vi "Lab Panel V5.31.vi"() -> ()   [LabVIEW 2017] (continued)
                            n1476 = local write "RESULT LAB04-1"(TRUE) -> ()
                            n1477 = local write "DISP LAB04-1"(w2766) -> ()
                          }
                        }
                      }
                      frame False {
                      }
                    }
                  }
                }
              }
              frame #7 {
                # "LAB04-2"
                n1478 = Equal?(x=w2769, y=2) -> (x = y?=w2772:bool)
                n1479 = local read "DISP LAB04-2"() -> (w2774:T4)
                n1480 = Unbundle(w2774) -> ("STATUS"=w2775:string)  [unwired: 2 out]
                n1481 = Equal?(x=w2775, y="RUN") -> (x = y?=w2771:bool)
                n1482 = And(x=w2771, y=w2772) -> (x .and. y?=w2770:bool)
                n1483 = case shown="True" w2770 {
                  tunnel: w2774 -> [_ w2778]
                  tunnel: w2768 -> [_ w2781]
                  frame False {
                  }
                  frame True {
                    n1484 = local read "SET LAB04-2"() -> (w2780:T5)
                    n1485 = local read "TDMS LAB04-2"() -> (w2777:refnum<k34>)
                    n1486 = Unbundle(w2778) -> ("CYCLE"=w2782:dbl)  [unwired: 2 out]
                    n1487 = Unbundle(w2780) -> ("T-RISE mins"=w2779:dbl)  [unwired: 4 out]
                    n1488 = Greater Or Equal?(x=w2782, y=w2781) -> (x >= y?=w2783:bool)
                    n1489 = case shown="True" w2783 {
                      tunnel: w2779 -> [w2786 _]
                      tunnel: w2778 -> [w2785 _]
                      tunnel: w2777 -> [w2784 _]
                      frame True {
                        n1490 = stacked-sequence {
                          tunnel: w2786 -> [w2789 _]
                          tunnel: w2785 -> [_ w2794]
                          tunnel: w2784 -> [w2787 _]
                          frame #0 {
                            n1491 = Build Array("T-RISE") -> (w2791:string[])
                            n1492 = Build Array(w2789) -> (w2790:dbl[])
                            n1493 = TDMS Write(0:w2787, 5:"TEST PASS", 7:w2791, 9:w2790) -> (15:w2793:errorcluster)  [unwired: 2 in, 3 out]
                            n1494 = local write "data file error"(w2793) -> ()
                          }
                          frame #1 {
                            n1495 = Bundle(cluster=w2794, "STATUS"="T-RISE PASS") -> (w2796:T4)  [unwired: 2 in]
                            n1496 = local write "RESULT LAB04-2"(TRUE) -> ()
                            n1497 = local write "DISP LAB04-2"(w2796) -> ()
                          }
                        }
                      }
                      frame False {
                      }
                    }
                  }
                }
              }
              frame #8 {
                # "LAB05-1"
                n1498 = Equal?(x=w2799, y=2) -> (x = y?=w2802:bool)
                n1499 = local read "DISP LAB05-1"() -> (w2804:T4)
                n1500 = Unbundle(w2804) -> ("STATUS"=w2805:string)  [unwired: 2 out]
                n1501 = Equal?(x=w2805, y="RUN") -> (x = y?=w2801:bool)
                n1502 = And(x=w2801, y=w2802) -> (x .and. y?=w2800:bool)
                n1503 = case shown="True" w2800 {
                  tunnel: w2804 -> [_ w2808]
                  tunnel: w2798 -> [_ w2811]
                  frame False {
                  }
                  frame True {
                    n1504 = local read "SET LAB05-1"() -> (w2810:T5)
                    n1505 = local read "TDMS LAB05-1"() -> (w2807:refnum<k34>)
                    n1506 = Unbundle(w2808) -> ("CYCLE"=w2812:dbl)  [unwired: 2 out]
                    n1507 = Unbundle(w2810) -> ("T-RISE mins"=w2809:dbl)  [unwired: 4 out]
                    n1508 = Greater Or Equal?(x=w2812, y=w2811) -> (x >= y?=w2813:bool)
                    n1509 = case shown="True" w2813 {
                      tunnel: w2809 -> [w2816 _]
                      tunnel: w2808 -> [w2815 _]
                      tunnel: w2807 -> [w2814 _]
                      frame True {
                        n1510 = stacked-sequence {
                          tunnel: w2816 -> [w2819 _]
                          tunnel: w2815 -> [_ w2824]
                          tunnel: w2814 -> [w2817 _]
                          frame #0 {
                            n1511 = Build Array("T-RISE") -> (w2821:string[])
                            n1512 = Build Array(w2819) -> (w2820:dbl[])
                            n1513 = TDMS Write(0:w2817, 5:"TEST PASS", 7:w2821, 9:w2820) -> (15:w2823:errorcluster)  [unwired: 2 in, 3 out]
                            n1514 = local write "data file error"(w2823) -> ()
                          }
                          frame #1 {
                            n1515 = Bundle(cluster=w2824, "STATUS"="T-RISE PASS") -> (w2826:T4)  [unwired: 2 in]
                            n1516 = local write "RESULT LAB05-1"(TRUE) -> ()
                            n1517 = local write "DISP LAB05-1"(w2826) -> ()
                          }
                        }
                      }
                      frame False {
                      }
                    }
                  }
                }
              }
              frame #9 {
                # "LAB05-2"
                n1518 = Equal?(x=w2829, y=2) -> (x = y?=w2832:bool)
                n1519 = local read "DISP LAB05-2"() -> (w2834:T4)
                n1520 = Unbundle(w2834) -> ("STATUS"=w2835:string)  [unwired: 2 out]
                n1521 = Equal?(x=w2835, y="RUN") -> (x = y?=w2831:bool)
                n1522 = And(x=w2831, y=w2832) -> (x .and. y?=w2830:bool)
                n1523 = case shown="True" w2830 {
                  tunnel: w2834 -> [_ w2838]
                  tunnel: w2828 -> [_ w2841]
                  frame False {
                  }
                  frame True {
                    n1524 = local read "SET LAB05-2"() -> (w2840:T5)
                    n1525 = local read "TDMS LAB05-2"() -> (w2837:refnum<k34>)
                    n1526 = Unbundle(w2838) -> ("CYCLE"=w2842:dbl)  [unwired: 2 out]
                    n1527 = Unbundle(w2840) -> ("T-RISE mins"=w2839:dbl)  [unwired: 4 out]
                    n1528 = Greater Or Equal?(x=w2842, y=w2841) -> (x >= y?=w2843:bool)
                    n1529 = case shown="True" w2843 {
                      tunnel: w2839 -> [w2846 _]
                      tunnel: w2838 -> [w2845 _]
                      tunnel: w2837 -> [w2844 _]
                      frame True {
                        n1530 = stacked-sequence {
                          tunnel: w2846 -> [w2849 _]
                          tunnel: w2845 -> [_ w2854]
                          tunnel: w2844 -> [w2847 _]
                          frame #0 {
                            n1531 = Build Array("T-RISE") -> (w2851:string[])
                            n1532 = Build Array(w2849) -> (w2850:dbl[])
                            n1533 = TDMS Write(0:w2847, 5:"TEST PASS", 7:w2851, 9:w2850) -> (15:w2853:errorcluster)  [unwired: 2 in, 3 out]
                            n1534 = local write "data file error"(w2853) -> ()
                          }
                          frame #1 {
                            n1535 = Bundle(cluster=w2854, "STATUS"="T-RISE PASS") -> (w2856:T4)  [unwired: 2 in]
                            n1536 = local write "RESULT LAB05-2"(TRUE) -> ()
                            n1537 = local write "DISP LAB05-2"(w2856) -> ()
                          }
                        }
                      }
                      frame False {
                      }
                    }
                  }
                }
              }
            }
          }
          frame #7 {
            # "Note : run lab0X-N. RUN LAB0X-N and O/I LAB0X-N   are written to digital I/O in frame 11"
            # "End test & close test files"
            n1538 = local read "MAIL SETTINGS"() -> (w2863:T8)
            n1539 = local read "TO (string):"() -> (w2858:string)
            n1540 = Unbundle(w2863) -> ("OUT SERVER ADDRESS"=w2862:string, "FROM ACCOUNT"=w2861:string)  [unwired: 5 out]
            n1541 = stacked-sequence {
              tunnel: w2873 -> [_ _ _ _ _ _ _ _ _ _]
              tunnel: w2874 -> [_ _ _ _ _ _ _ _ _ _]
              tunnel: w2872 -> [_ _ _ _ _ _ _ _ _ _]
              tunnel: w2871 -> [_ _ _ _ _ _ _ _ _ _]
              tunnel: w2870 -> [_ _ _ _ _ _ _ _ _ _]
              tunnel: w2869 -> [_ _ _ _ _ _ _ _ _ _]
              tunnel: w2868 -> [_ _ _ _ _ _ _ _ _ _]
              tunnel: w2867 -> [_ _ _ _ _ _ _ _ _ _]
              tunnel: w2866 -> [_ _ _ _ _ _ _ _ _ _]
              tunnel: w2865 -> [_ _ _ _ _ _ _ _ _ _]
              tunnel: w2862 -> [w2879 w2931 w2979 w3026 w3073 w3120 w3167 w3214 w3261 w3308]
              tunnel: w2861 -> [w2878 w2930 w2978 w3025 w3072 w3119 w3166 w3213 w3260 w3307]
              tunnel: "Mail Test File To:" -> [w2877 w2929 w2977 w3024 w3071 w3118 w3165 w3212 w3259 w3306]
              tunnel: "Mail Test Fail" -> [w2876 w2928 w2976 w3023 w3070 w3117 w3164 w3211 w3258 w3305]
              frame #0 {
                # "LAB01-1"
                n1542 = local read "DISP LAB01-1"() -> (w2875:T4)
                n1543 = global write "Global display 2.vi" "DISP LAB01-1"(w2875) -> ()
                n1544 = local read "run lab01-1"() -> (w2880:bool)
                n1545 = local read "TDMS LAB01-1"() -> (w2881:refnum<k34>)
                n1546 = Unbundle(w2875) -> ("CYCLE"=w2883:dbl, "STATUS"=w2882:string)  [unwired: 1 out]
                n1547 = case shown="True" w2880 {
                  tunnel: w2883 -> [_ w2889]
                  tunnel: w2875 -> [_ w2891]
                  tunnel: w2882 -> [_ w2888]
                  tunnel: w2881 -> [_ w2890]
                  tunnel: w2879 -> [_ w2887]
                  tunnel: w2878 -> [_ w2886]
                  tunnel: w2877 -> [_ w2885]
                  tunnel: w2876 -> [_ w2884]
                  frame False {
                  }
                  frame True {
                    n1548 = Not Equal?(x=w2888, y="RUN") -> (x != y?=w2892:bool)
                    n1549 = Greater?(x=w2889, y=2.0) -> (0:w2894:bool)
                    n1550 = And(x=w2894, y=w2892) -> (x .and. y?=w2893:bool)
                    n1551 = case shown="True" w2893 {
                      tunnel: w2891 -> [_ w2904]
                      tunnel: w2890 -> [_ w2903]
                      tunnel: w2889 -> [_ w2902]
                      tunnel: w2888 -> [_ w2901]
                      tunnel: w2887 -> [_ w2900]
                      tunnel: w2886 -> [_ w2899]
                      tunnel: w2885 -> [_ w2898]
                      tunnel: w2884 -> [_ w2897]
                      frame False {
                      }
                      frame True {
                        n1552 = stacked-sequence {
                          tunnel: w2904 -> [w2908 _ _]
                          tunnel: w2903 -> [_ w2910 _]
                          tunnel: w2902 -> [_ _ _]
                          tunnel: w2901 -> [_ _ w2916]
                          tunnel: w2900 -> [_ _ w2915]
                          tunnel: w2899 -> [_ _ w2914]
                          tunnel: w2898 -> [_ _ w2913]
                          tunnel: w2897 -> [_ _ w2912]
                          frame #0 {
                            w2905 = FALSE
                            n1553 = local write "mail control"("END") -> ()
                            n1554 = Bundle(cluster=w2908) -> (w2907:T4)  [unwired: 3 in]
                            n1555 = local write "DISP LAB01-1"(w2907) -> ()
                            n1556 = local write "O/I  LAB01-1"(w2905) -> ()
                            n1557 = local write "run lab01-1"(w2905) -> ()
                            n1558 = local write "RUN LAB01-1"(w2905) -> ()
                          }
                          frame #1 {
                            n1559 = TDMS Close(11:w2910) -> (0:w2909:errorcluster)  [unwired: 1 in, 1 out]
                            n1560 = local write "data file error"(w2909) -> ()
                          }
                          frame #2 {
                            n1561 = stacked-sequence {
                              tunnel: "LAB01-1" -> [w2918 w2921 _]
                              tunnel: w2916 -> [_ w2927 _]
                              tunnel: w2915 -> [_ w2926 _]
                              tunnel: w2914 -> [_ w2925 _]
                              tunnel: w2913 -> [_ w2924 _]
                              tunnel: w2912 -> [_ w2923 _]
                              frame #0 {
                                n1562 = call "sub vi - defrag tdms v1.vi"("panel id"=w2918) -> ("error out"=w2917:errorcluster)  [unwired: 10 in]
                                n1563 = local write "data file error"(w2917) -> ()
                              }
                              frame #1 {
                                n1564 = Bundle By Name(cluster=T23 {"status"="", "mail server"="", "mail from"="", "mail to"="", "mail file"=FALSE} ("Input Cluster"), "status"=w2927, "mail server"=w2926, "mail from"=w2925, "mail to"=w2924, "mail file"=w2923) -> (w2920:T23)
                                n1565 = call "Save data file (pass-fail) v5.vi"("Input Cluster"=w2920, "panel id"=w2921) -> ("network file save error"=w2922:errorcluster)  [unwired: 8 in, 1 out]
                                n1566 = local write "data file error"(w2922) -> ()
                              }
                              frame #2 {
                              }
                            }
                          }
                        }
                      }
                    }
                  }
                }
              }
              frame #1 {
                # "LAB01-2"
                n1567 = local read "run lab01-2"() -> (w2932:bool)
                n1568 = case shown="True" w2932 {
                  tunnel: w2931 -> [_ w2937]
                  tunnel: w2930 -> [_ w2936]
                  tunnel: w2929 -> [_ w2935]
                  tunnel: w2928 -> [_ w2934]
                  frame False {
                  }
                  frame True {
                    n1569 = local read "DISP LAB01-2"() -> (w2933:T4)
                    n1570 = global write "Global display 2.vi" "DISP LAB01-2"(w2933) -> ()
                    n1571 = local read "TDMS LAB01-2"() -> (w2944:refnum<k34>)
                    n1572 = Unbundle(w2933) -> ("CYCLE"=w2939:dbl, "STATUS"=w2938:string)  [unwired: 1 out]
                    n1573 = Not Equal?(x=w2938, y="RUN") -> (x != y?=w2941:bool)
                    n1574 = Greater?(x=w2939, y=2.0) -> (0:w2942:bool)
                    n1575 = And(x=w2942, y=w2941) -> (x .and. y?=w2940:bool)
                    n1576 = case shown="True" w2940 {
                      tunnel: w2933 -> [_ w2953]
                      tunnel: w2944 -> [_ w2952]
                      tunnel: w2939 -> [_ w2951]
                      tunnel: w2938 -> [_ w2950]
                      tunnel: w2937 -> [_ w2949]
                      tunnel: w2936 -> [_ w2948]
                      tunnel: w2935 -> [_ w2947]
                      tunnel: w2934 -> [_ w2946]
                      frame False {
                      }
                      frame True {
                        n1577 = stacked-sequence {
                          tunnel: w2953 -> [w2956 _ _]
                          tunnel: w2952 -> [_ w2958 _]
                          tunnel: w2951 -> [_ _ _]
                          tunnel: w2950 -> [_ _ w2964]
                          tunnel: w2949 -> [_ _ w2963]
                          tunnel: w2948 -> [_ _ w2962]
                          tunnel: w2947 -> [_ _ w2961]
                          tunnel: w2946 -> [_ _ w2960]
                          frame #0 {
                            w2954 = FALSE
                            n1578 = local write "mail control"("END") -> ()
                            n1579 = Bundle(cluster=w2956) -> (w2957:T4)  [unwired: 3 in]
                            n1580 = local write "RUN LAB01-2"(w2954) -> ()
                            n1581 = local write "run lab01-2"(w2954) -> ()
                            n1582 = local write "O/I  LAB01-2"(w2954) -> ()
                            n1583 = local write "DISP LAB01-2"(w2957) -> ()
                          }
                          frame #1 {
                            n1584 = TDMS Close(11:w2958) -> (0:w2959:errorcluster)  [unwired: 1 in, 1 out]
                            n1585 = local write "data file error"(w2959) -> ()
                          }
                          frame #2 {
                            n1586 = stacked-sequence {
                              tunnel: "LAB01-2" -> [w2967 w2968]
                              tunnel: w2964 -> [_ w2973]
                              tunnel: w2963 -> [_ w2972]
                              tunnel: w2962 -> [_ w2971]
                              tunnel: w2961 -> [_ w2970]
                              tunnel: w2960 -> [_ w2969]
                              frame #0 {
                                n1587 = call "sub vi - defrag tdms v1.vi"("panel id"=w2967) -> ("error out"=w2966:errorcluster)  [unwired: 10 in]
                                n1588 = local write "data file error"(w2966) -> ()
                              }
                              frame #1 {
                                n1589 = Bundle("STATUS"=w2973, "OUT SERVER ADDRESS"=w2972, "FROM ACCOUNT"=w2971, "Mail Test File To:"=w2970, "Mail Test Fail"=w2969) -> (w2975:T29)  [unwired: 1 in]
                                n1590 = call "Save data file (pass-fail) v5.vi"("Input Cluster"=w2975, "panel id"=w2968) -> ("network file save error"=w2974:errorcluster)  [unwired: 8 in, 1 out]
                                n1591 = local write "data file error"(w2974) -> ()
                              }
                            }
                          }
                        }
                      }
                    }
                  }
                }
              }
              frame #2 {
                # "LAB02-1"
                n1592 = local read "run lab02-1"() -> (w2980:bool)
                n1593 = case shown="True" w2980 {
                  tunnel: w2979 -> [_ w2985]
                  tunnel: w2978 -> [_ w2984]
                  tunnel: w2977 -> [_ w2983]
                  tunnel: w2976 -> [_ w2982]
                  frame False {
                  }
                  frame True {
                    n1594 = local read "DISP LAB02-1"() -> (w2981:T4)
                    n1595 = global write "Global display 2.vi" "DISP LAB02-1"(w2981) -> ()
                    n1596 = Unbundle(w2981) -> ("CYCLE"=w2989:dbl, "STATUS"=w2986:string)  [unwired: 1 out]
                    n1597 = local read "TDMS LAB02-1"() -> (w2992:refnum<k34>)
                    n1598 = Not Equal?(x=w2986, y="RUN") -> (x != y?=w2988:bool)
                    n1599 = Greater?(x=w2989, y=2.0) -> (0:w2990:bool)
                    n1600 = And(x=w2990, y=w2988) -> (x .and. y?=w2987:bool)
                    n1601 = case shown="True" w2987 {
                      tunnel: w2981 -> [_ w3000]
                      tunnel: w2992 -> [_ w2999]
                      tunnel: w2986 -> [_ w2998]
                      tunnel: w2985 -> [_ w2997]
                      tunnel: w2984 -> [_ w2996]
                      tunnel: w2983 -> [_ w2995]
                      tunnel: w2982 -> [_ w2994]
                      frame False {
                      }
                      frame True {
                        n1602 = stacked-sequence {
                          tunnel: w3000 -> [w3003 _ _]
                          tunnel: w2999 -> [_ w3005 _]
                          tunnel: w2998 -> [_ _ w3011]
                          tunnel: w2997 -> [_ _ w3010]
                          tunnel: w2996 -> [_ _ w3009]
                          tunnel: w2995 -> [_ _ w3008]
                          tunnel: w2994 -> [_ _ w3007]
                          frame #0 {
                            w3001 = FALSE
                            n1603 = local write "mail control"("END") -> ()
                            n1604 = Bundle(cluster=w3003) -> (w3004:T4)  [unwired: 3 in]
                            n1605 = local write "O/I  LAB02-1"(w3001) -> ()
                            n1606 = local write "RUN LAB02-1"(w3001) -> ()
                            n1607 = local write "run lab02-1"(w3001) -> ()
                            n1608 = local write "DISP LAB02-1"(w3004) -> ()
                          }
                          frame #1 {
                            n1609 = TDMS Close(11:w3005) -> (0:w3006:errorcluster)  [unwired: 1 in, 1 out]
                            n1610 = local write "data file error"(w3006) -> ()
                          }
                          frame #2 {
                            n1611 = stacked-sequence {
                              tunnel: "LAB02-1" -> [w3014 w3021]
                              tunnel: w3011 -> [_ w3019]
                              tunnel: w3010 -> [_ w3018]
                              tunnel: w3009 -> [_ w3017]
                              tunnel: w3008 -> [_ w3016]
                              tunnel: w3007 -> [_ w3015]
                              frame #0 {
                                n1612 = call "sub vi - defrag tdms v1.vi"("panel id"=w3014) -> ("error out"=w3013:errorcluster)  [unwired: 10 in]
                                n1613 = local write "data file error"(w3013) -> ()
                              }
                              frame #1 {
                                n1614 = Bundle("STATUS"=w3019, "OUT SERVER ADDRESS"=w3018, "FROM ACCOUNT"=w3017, "Mail Test File To:"=w3016, "Mail Test Fail"=w3015) -> (w3020:T29)  [unwired: 1 in]
                                n1615 = call "Save data file (pass-fail) v5.vi"("Input Cluster"=w3020, "panel id"=w3021) -> ("network file save error"=w3022:errorcluster)  [unwired: 8 in, 1 out]
                                n1616 = local write "data file error"(w3022) -> ()
                              }
                            }
                          }
                        }
                      }
                    }
                  }
                }
              }
              frame #3 {
                # "LAB02-2"
                n1617 = local read "run lab02-2"() -> (w3027:bool)
                n1618 = case shown="True" w3027 {
                  tunnel: w3026 -> [_ w3033]
                  tunnel: w3025 -> [_ w3032]
                  tunnel: w3024 -> [_ w3031]
                  tunnel: w3023 -> [_ w3030]
                  frame False {
                  }
                  frame True {
                    n1619 = local read "DISP LAB02-2"() -> (w3029:T4)
                    n1620 = global write "Global display 2.vi" "DISP LAB02-2"(w3029) -> ()
                    n1621 = local read "TDMS LAB02-2"() -> (w3039:refnum<k34>)
                    n1622 = Unbundle(w3029) -> ("CYCLE"=w3028:dbl, "STATUS"=w3034:string)  [unwired: 1 out]
                    n1623 = Not Equal?(x=w3034, y="RUN") -> (x != y?=w3036:bool)
                    n1624 = Greater?(x=w3028, y=2.0) -> (0:w3037:bool)
                    n1625 = And(x=w3037, y=w3036) -> (x .and. y?=w3035:bool)
                    n1626 = case shown="True" w3035 {
                      tunnel: w3029 -> [_ w3047]
                      tunnel: w3039 -> [_ w3046]
                      tunnel: w3034 -> [_ w3045]
                      tunnel: w3033 -> [_ w3044]
                      tunnel: w3032 -> [_ w3043]
                      tunnel: w3031 -> [_ w3042]
                      tunnel: w3030 -> [_ w3041]
                      frame False {
                      }
                      frame True {
                        n1627 = stacked-sequence {
                          tunnel: w3047 -> [w3050 _ _]
                          tunnel: w3046 -> [_ w3052 _]
                          tunnel: w3045 -> [_ _ w3058]
                          tunnel: w3044 -> [_ _ w3057]
                          tunnel: w3043 -> [_ _ w3056]
                          tunnel: w3042 -> [_ _ w3055]
                          tunnel: w3041 -> [_ _ w3054]
                          frame #0 {
                            w3048 = FALSE
                            n1628 = local write "mail control"("END") -> ()
                            n1629 = Bundle(cluster=w3050) -> (w3051:T4)  [unwired: 3 in]
                            n1630 = local write "O/I  LAB02-2"(w3048) -> ()
                            n1631 = local write "run lab02-2"(w3048) -> ()
                            n1632 = local write "RUN LAB02-2"(w3048) -> ()
                            n1633 = local write "DISP LAB02-2"(w3051) -> ()
                          }
                          frame #1 {
                            n1634 = TDMS Close(11:w3052) -> (0:w3053:errorcluster)  [unwired: 1 in, 1 out]
                            n1635 = local write "data file error"(w3053) -> ()
                          }
                          frame #2 {
                            n1636 = stacked-sequence {
                              tunnel: "LAB02-2" -> [w3061 w3067]
                              tunnel: w3058 -> [_ w3066]
                              tunnel: w3057 -> [_ w3065]
                              tunnel: w3056 -> [_ w3064]
                              tunnel: w3055 -> [_ w3063]
                              tunnel: w3054 -> [_ w3062]
                              frame #0 {
                                n1637 = call "sub vi - defrag tdms v1.vi"("panel id"=w3061) -> ("error out"=w3060:errorcluster)  [unwired: 10 in]
                                n1638 = local write "data file error"(w3060) -> ()
                              }
                              frame #1 {
                                n1639 = Bundle("STATUS"=w3066, "OUT SERVER ADDRESS"=w3065, "FROM ACCOUNT"=w3064, "Mail Test File To:"=w3063, "Mail Test Fail"=w3062) -> (w3069:T29)  [unwired: 1 in]
                                n1640 = call "Save data file (pass-fail) v5.vi"("Input Cluster"=w3069, "panel id"=w3067) -> ("network file save error"=w3068:errorcluster)  [unwired: 8 in, 1 out]
                                n1641 = local write "data file error"(w3068) -> ()
                              }
                            }
                          }
                        }
                      }
                    }
                  }
                }
              }
              frame #4 {
                # "LAB03-1"
                n1642 = local read "run lab03-1"() -> (w3074:bool)
                n1643 = case shown="True" w3074 {
                  tunnel: w3073 -> [_ w3079]
                  tunnel: w3072 -> [_ w3078]
                  tunnel: w3071 -> [_ w3077]
                  tunnel: w3070 -> [_ w3076]
                  frame False {
                  }
                  frame True {
                    n1644 = local read "DISP LAB03-1"() -> (w3075:T4)
                    n1645 = local read "TDMS LAB03-1"() -> (w3086:refnum<k34>)
                    n1646 = global write "Global display 2.vi" "DISP LAB03-1"(w3075) -> ()
                    n1647 = Unbundle(w3075) -> ("CYCLE"=w3083:dbl, "STATUS"=w3080:string)  [unwired: 1 out]
                    n1648 = Not Equal?(x=w3080, y="RUN") -> (x != y?=w3082:bool)
                    n1649 = Greater?(x=w3083, y=2.0) -> (0:w3084:bool)
                    n1650 = And(x=w3084, y=w3082) -> (x .and. y?=w3081:bool)
                    n1651 = case shown="True" w3081 {
                      tunnel: w3075 -> [_ w3094]
                      tunnel: w3086 -> [_ w3093]
                      tunnel: w3080 -> [_ w3092]
                      tunnel: w3079 -> [_ w3091]
                      tunnel: w3078 -> [_ w3090]
                      tunnel: w3077 -> [_ w3089]
                      tunnel: w3076 -> [_ w3088]
                      frame False {
                      }
                      frame True {
                        n1652 = stacked-sequence {
                          tunnel: w3094 -> [w3097 _ _]
                          tunnel: w3093 -> [_ w3099 _]
                          tunnel: w3092 -> [_ _ w3105]
                          tunnel: w3091 -> [_ _ w3104]
                          tunnel: w3090 -> [_ _ w3103]
                          tunnel: w3089 -> [_ _ w3102]
                          tunnel: w3088 -> [_ _ w3101]
                          frame #0 {
                            w3095 = FALSE
                            n1653 = local write "mail control"("END") -> ()
                            n1654 = Bundle(cluster=w3097) -> (w3098:T4)  [unwired: 3 in]
                            n1655 = local write "O/I  LAB03-1"(w3095) -> ()
                            n1656 = local write "run lab03-1"(w3095) -> ()
                            n1657 = local write "RUN LAB03-1"(w3095) -> ()
                            n1658 = local write "DISP LAB03-1"(w3098) -> ()
                          }
                          frame #1 {
                            n1659 = TDMS Close(11:w3099) -> (0:w3100:errorcluster)  [unwired: 1 in, 1 out]
                            n1660 = local write "data file error"(w3100) -> ()
                          }
                          frame #2 {
                            n1661 = stacked-sequence {
                              tunnel: "LAB03-1" -> [w3108 w3114]
                              tunnel: w3105 -> [_ w3113]
                              tunnel: w3104 -> [_ w3112]
                              tunnel: w3103 -> [_ w3111]
                              tunnel: w3102 -> [_ w3110]
                              tunnel: w3101 -> [_ w3109]
                              frame #0 {
                                n1662 = call "sub vi - defrag tdms v1.vi"("panel id"=w3108) -> ("error out"=w3107:errorcluster)  [unwired: 10 in]
                                n1663 = local write "data file error"(w3107) -> ()
                              }
                              frame #1 {
                                n1664 = Bundle("STATUS"=w3113, "OUT SERVER ADDRESS"=w3112, "FROM ACCOUNT"=w3111, "Mail Test File To:"=w3110, "Mail Test Fail"=w3109) -> (w3116:T29)  [unwired: 1 in]
                                n1665 = call "Save data file (pass-fail) v5.vi"("Input Cluster"=w3116, "panel id"=w3114) -> ("network file save error"=w3115:errorcluster)  [unwired: 8 in, 1 out]
                                n1666 = local write "data file error"(w3115) -> ()
                              }
                            }
                          }
                        }
                      }
                    }
                  }
                }
              }
              frame #5 {
                # "LAB03-2"
                n1667 = local read "run lab03-2"() -> (w3121:bool)
                n1668 = case shown="True" w3121 {
                  tunnel: w3120 -> [_ w3126]
                  tunnel: w3119 -> [_ w3125]
                  tunnel: w3118 -> [_ w3124]
                  tunnel: w3117 -> [_ w3123]
                  frame False {
                  }
                  frame True {
                    n1669 = local read "DISP LAB03-2"() -> (w3122:T4)
                    n1670 = global write "Global display 2.vi" "DISP LAB03-2"(w3122) -> ()
                    n1671 = Unbundle(w3122) -> ("CYCLE"=w3130:dbl, "STATUS"=w3127:string)  [unwired: 1 out]
                    n1672 = local read "TDMS LAB03-2"() -> (w3133:refnum<k34>)
                    n1673 = Not Equal?(x=w3127, y="RUN") -> (x != y?=w3129:bool)
                    n1674 = Greater?(x=w3130, y=2.0) -> (0:w3131:bool)
                    n1675 = And(x=w3131, y=w3129) -> (x .and. y?=w3128:bool)
                    n1676 = case shown="True" w3128 {
                      tunnel: w3122 -> [_ w3141]
                      tunnel: w3133 -> [_ w3140]
                      tunnel: w3127 -> [_ w3139]
                      tunnel: w3126 -> [_ w3138]
                      tunnel: w3125 -> [_ w3137]
                      tunnel: w3124 -> [_ w3136]
                      tunnel: w3123 -> [_ w3135]
                      frame False {
                      }
                      frame True {
                        n1677 = stacked-sequence {
                          tunnel: w3141 -> [w3144 _ _]
                          tunnel: w3140 -> [_ w3146 _]
                          tunnel: w3139 -> [_ _ w3152]
                          tunnel: w3138 -> [_ _ w3151]
                          tunnel: w3137 -> [_ _ w3150]
                          tunnel: w3136 -> [_ _ w3149]
                          tunnel: w3135 -> [_ _ w3148]
                          frame #0 {
                            w3142 = FALSE
                            n1678 = local write "mail control"("END") -> ()
                            n1679 = Bundle(cluster=w3144) -> (w3145:T4)  [unwired: 3 in]
                            n1680 = local write "RUN LAB03-2"(w3142) -> ()
                            n1681 = local write "O/I  LAB03-2"(w3142) -> ()
                            n1682 = local write "DISP LAB03-2"(w3145) -> ()
                            n1683 = local write "run lab03-2"(w3142) -> ()
                          }
                          frame #1 {
                            n1684 = TDMS Close(11:w3146) -> (0:w3147:errorcluster)  [unwired: 1 in, 1 out]
                            n1685 = local write "data file error"(w3147) -> ()
                          }
                          frame #2 {
                            n1686 = stacked-sequence {
                              tunnel: "LAB03-2" -> [w3155 w3156]
                              tunnel: w3152 -> [_ w3161]
                              tunnel: w3151 -> [_ w3160]
                              tunnel: w3150 -> [_ w3159]
                              tunnel: w3149 -> [_ w3158]
                              tunnel: w3148 -> [_ w3157]
                              frame #0 {
                                n1687 = call "sub vi - defrag tdms v1.vi"("panel id"=w3155) -> ("error out"=w3154:errorcluster)  [unwired: 10 in]
                                n1688 = local write "data file error"(w3154) -> ()
                              }
                              frame #1 {
                                n1689 = Bundle("STATUS"=w3161, "OUT SERVER ADDRESS"=w3160, "FROM ACCOUNT"=w3159, "Mail Test File To:"=w3158, "Mail Test Fail"=w3157) -> (w3163:T29)  [unwired: 1 in]
                                n1690 = call "Save data file (pass-fail) v5.vi"("Input Cluster"=w3163, "panel id"=w3156) -> ("network file save error"=w3162:errorcluster)  [unwired: 8 in, 1 out]
                                n1691 = local write "data file error"(w3162) -> ()
                              }
                            }
                          }
                        }
                      }
                    }
                  }
                }
              }
              frame #6 {
                # "LAB04-1"
                n1692 = local read "run lab04-1"() -> (w3168:bool)
                n1693 = case shown="True" w3168 {
                  tunnel: w3167 -> [_ w3173]
                  tunnel: w3166 -> [_ w3172]
                  tunnel: w3165 -> [_ w3171]
                  tunnel: w3164 -> [_ w3170]
                  frame False {
                  }
                  frame True {
                    n1694 = local read "DISP LAB04-1"() -> (w3169:T4)
                    n1695 = Unbundle(w3169) -> ("CYCLE"=w3177:dbl, "STATUS"=w3174:string)  [unwired: 1 out]
                    n1696 = local read "TDMS LAB04-1"() -> (w3180:refnum<k34>)
                    n1697 = global write "Global display 2.vi" "DISP LAB04-1"(w3169) -> ()
                    n1698 = Not Equal?(x=w3174, y="RUN") -> (x != y?=w3176:bool)
                    n1699 = Greater?(x=w3177, y=2.0) -> (0:w3178:bool)
                    n1700 = And(x=w3178, y=w3176) -> (x .and. y?=w3175:bool)
                    n1701 = case shown="True" w3175 {
                      tunnel: w3169 -> [_ w3188]
                      tunnel: w3180 -> [_ w3187]
                      tunnel: w3174 -> [_ w3186]
                      tunnel: w3173 -> [_ w3185]
                      tunnel: w3172 -> [_ w3184]
                      tunnel: w3171 -> [_ w3183]
                      tunnel: w3170 -> [_ w3182]
                      frame False {
                      }
                      frame True {
                        n1702 = stacked-sequence {
                          tunnel: w3188 -> [w3191 _ _]
                          tunnel: w3187 -> [_ w3193 _]
                          tunnel: w3186 -> [_ _ w3199]
                          tunnel: w3185 -> [_ _ w3198]
                          tunnel: w3184 -> [_ _ w3197]
                          tunnel: w3183 -> [_ _ w3196]
                          tunnel: w3182 -> [_ _ w3195]
                          frame #0 {
                            w3189 = FALSE
                            n1703 = local write "mail control"("END") -> ()
                            n1704 = Bundle(cluster=w3191) -> (w3192:T4)  [unwired: 3 in]
                            n1705 = local write "RUN LAB04-1"(w3189) -> ()
                            n1706 = local write "O/I  LAB04-1"(w3189) -> ()
                            n1707 = local write "run lab04-1"(w3189) -> ()
                            n1708 = local write "DISP LAB04-1"(w3192) -> ()
                          }
                          frame #1 {
                            n1709 = TDMS Close(11:w3193) -> (0:w3194:errorcluster)  [unwired: 1 in, 1 out]
                            n1710 = local write "data file error"(w3194) -> ()
                          }
                          frame #2 {
                            n1711 = stacked-sequence {
                              tunnel: "LAB04-1" -> [w3202 w3203]
                              tunnel: w3199 -> [_ w3208]
                              tunnel: w3198 -> [_ w3207]
                              tunnel: w3197 -> [_ w3206]
                              tunnel: w3196 -> [_ w3205]
                              tunnel: w3195 -> [_ w3204]
                              frame #0 {
                                n1712 = call "sub vi - defrag tdms v1.vi"("panel id"=w3202) -> ("error out"=w3201:errorcluster)  [unwired: 10 in]
                                n1713 = local write "data file error"(w3201) -> ()
                              }
                              frame #1 {
                                n1714 = Bundle("STATUS"=w3208, "OUT SERVER ADDRESS"=w3207, "FROM ACCOUNT"=w3206, "Mail Test File To:"=w3205, "Mail Test Fail"=w3204) -> (w3210:T29)  [unwired: 1 in]
                                n1715 = call "Save data file (pass-fail) v5.vi"("Input Cluster"=w3210, "panel id"=w3203) -> ("network file save error"=w3209:errorcluster)  [unwired: 8 in, 1 out]
                                n1716 = local write "data file error"(w3209) -> ()
                              }
                            }
                          }
                        }
                      }
                    }
                  }
                }
              }
              frame #7 {
                # "LAB04-2"
                n1717 = local read "run lab04-2"() -> (w3215:bool)
                n1718 = case shown="True" w3215 {
                  tunnel: w3214 -> [_ w3220]
                  tunnel: w3213 -> [_ w3219]
                  tunnel: w3212 -> [_ w3218]
                  tunnel: w3211 -> [_ w3217]
                  frame False {
                  }
                  frame True {
                    n1719 = local read "DISP LAB04-2"() -> (w3216:T4)
                    n1720 = Unbundle(w3216) -> ("CYCLE"=w3224:dbl, "STATUS"=w3221:string)  [unwired: 1 out]
                    n1721 = global write "Global display 2.vi" "DISP LAB04-2"(w3216) -> ()
                    n1722 = Not Equal?(x=w3221, y="RUN") -> (x != y?=w3223:bool)
                    n1723 = local read "TDMS LAB04-2"() -> (w3227:refnum<k34>)
                    n1724 = Greater?(x=w3224, y=2.0) -> (0:w3225:bool)
                    n1725 = And(x=w3225, y=w3223) -> (x .and. y?=w3222:bool)
                    n1726 = case shown="True" w3222 {
                      tunnel: w3216 -> [_ w3235]
                      tunnel: w3227 -> [_ w3234]
                      tunnel: w3221 -> [_ w3233]
                      tunnel: w3220 -> [_ w3232]
                      tunnel: w3219 -> [_ w3231]
                      tunnel: w3218 -> [_ w3230]
                      tunnel: w3217 -> [_ w3229]
                      frame False {
                      }
                      frame True {
                        n1727 = stacked-sequence {
                          tunnel: w3235 -> [w3238 _ _]
                          tunnel: w3234 -> [_ w3240 _]
                          tunnel: w3233 -> [_ _ w3246]
                          tunnel: w3232 -> [_ _ w3245]
                          tunnel: w3231 -> [_ _ w3244]
                          tunnel: w3230 -> [_ _ w3243]
                          tunnel: w3229 -> [_ _ w3242]
                          frame #0 {
                            w3236 = FALSE
                            n1728 = local write "mail control"("END") -> ()
                            n1729 = Bundle(cluster=w3238) -> (w3239:T4)  [unwired: 3 in]
                            n1730 = local write "O/I  LAB04-2"(w3236) -> ()
                            n1731 = local write "RUN LAB04-2"(w3236) -> ()
                            n1732 = local write "run lab04-2"(w3236) -> ()
                            n1733 = local write "DISP LAB04-2"(w3239) -> ()
                          }
                          frame #1 {
                            n1734 = TDMS Close(11:w3240) -> (0:w3241:errorcluster)  [unwired: 1 in, 1 out]
                            n1735 = local write "data file error"(w3241) -> ()
                          }
                          frame #2 {
                            n1736 = stacked-sequence {
                              tunnel: "LAB04-2" -> [w3249 w3250]
                              tunnel: w3246 -> [_ w3255]
                              tunnel: w3245 -> [_ w3254]
                              tunnel: w3244 -> [_ w3253]
                              tunnel: w3243 -> [_ w3252]
                              tunnel: w3242 -> [_ w3251]
                              frame #0 {
                                n1737 = call "sub vi - defrag tdms v1.vi"("panel id"=w3249) -> ("error out"=w3248:errorcluster)  [unwired: 10 in]
                                n1738 = local write "data file error"(w3248) -> ()
                              }
                              frame #1 {
                                n1739 = Bundle("STATUS"=w3255, "OUT SERVER ADDRESS"=w3254, "FROM ACCOUNT"=w3253, "Mail Test File To:"=w3252, "Mail Test Fail"=w3251) -> (w3257:T29)  [unwired: 1 in]
                                n1740 = call "Save data file (pass-fail) v5.vi"("Input Cluster"=w3257, "panel id"=w3250) -> ("network file save error"=w3256:errorcluster)  [unwired: 8 in, 1 out]
                                n1741 = local write "data file error"(w3256) -> ()
                              }
                            }
                          }
                        }
                      }
                    }
                  }
                }
              }
              frame #8 {
                # "LAB05-1"
                n1742 = local read "run lab05-1"() -> (w3262:bool)
                n1743 = case shown="True" w3262 {
                  tunnel: w3261 -> [_ w3267]
                  tunnel: w3260 -> [_ w3266]
                  tunnel: w3259 -> [_ w3265]
                  tunnel: w3258 -> [_ w3264]
                  frame False {
                  }
                  frame True {
                    n1744 = local read "DISP LAB05-1"() -> (w3263:T4)
                    n1745 = Unbundle(w3263) -> ("CYCLE"=w3271:dbl, "STATUS"=w3268:string)  [unwired: 1 out]
                    n1746 = global write "Global display 2.vi" "DISP LAB05-1"(w3263) -> ()
                    n1747 = Not Equal?(x=w3268, y="RUN") -> (x != y?=w3270:bool)
                    n1748 = local read "TDMS LAB05-1"() -> (w3274:refnum<k34>)
                    n1749 = Greater?(x=w3271, y=2.0) -> (0:w3272:bool)
                    n1750 = And(x=w3272, y=w3270) -> (x .and. y?=w3269:bool)
                    n1751 = case shown="True" w3269 {
                      tunnel: w3263 -> [_ w3282]
                      tunnel: w3274 -> [_ w3281]
                      tunnel: w3268 -> [_ w3280]
                      tunnel: w3267 -> [_ w3279]
                      tunnel: w3266 -> [_ w3278]
                      tunnel: w3265 -> [_ w3277]
                      tunnel: w3264 -> [_ w3276]
                      frame False {
                      }
                      frame True {
                        n1752 = stacked-sequence {
                          tunnel: w3282 -> [w3285 _ _]
                          tunnel: w3281 -> [_ w3287 _]
                          tunnel: w3280 -> [_ _ w3293]
                          tunnel: w3279 -> [_ _ w3292]
                          tunnel: w3278 -> [_ _ w3291]
                          tunnel: w3277 -> [_ _ w3290]
                          tunnel: w3276 -> [_ _ w3289]
                          frame #0 {
                            w3283 = FALSE
                            n1753 = local write "mail control"("END") -> ()
                            n1754 = Bundle(cluster=w3285) -> (w3286:T4)  [unwired: 3 in]
                            n1755 = local write "O/I  LAB05-1"(w3283) -> ()
                            n1756 = local write "RUN LAB05-1"(w3283) -> ()
                            n1757 = local write "run lab05-1"(w3283) -> ()
                            n1758 = local write "DISP LAB05-1"(w3286) -> ()
                          }
                          frame #1 {
                            n1759 = TDMS Close(11:w3287) -> (0:w3288:errorcluster)  [unwired: 1 in, 1 out]
                            n1760 = local write "data file error"(w3288) -> ()
                          }
                          frame #2 {
                            n1761 = stacked-sequence {
                              tunnel: "LAB05-1" -> [w3296 w3302]
                              tunnel: w3293 -> [_ w3301]
                              tunnel: w3292 -> [_ w3300]
                              tunnel: w3291 -> [_ w3299]
                              tunnel: w3290 -> [_ w3298]
                              tunnel: w3289 -> [_ w3297]
                              frame #0 {
                                n1762 = call "sub vi - defrag tdms v1.vi"("panel id"=w3296) -> ("error out"=w3295:errorcluster)  [unwired: 10 in]
                                n1763 = local write "data file error"(w3295) -> ()
                              }
                              frame #1 {
                                n1764 = Bundle("STATUS"=w3301, "OUT SERVER ADDRESS"=w3300, "FROM ACCOUNT"=w3299, "Mail Test File To:"=w3298, "Mail Test Fail"=w3297) -> (w3304:T29)  [unwired: 1 in]
                                n1765 = call "Save data file (pass-fail) v5.vi"("Input Cluster"=w3304, "panel id"=w3302) -> ("network file save error"=w3303:errorcluster)  [unwired: 8 in, 1 out]
                                n1766 = local write "data file error"(w3303) -> ()
                              }
                            }
                          }
                        }
                      }
                    }
                  }
                }
              }
              frame #9 {
                # "LAB05-2"
                n1767 = local read "run lab05-2"() -> (w3309:bool)
                n1768 = case shown="True" w3309 {
                  tunnel: w3308 -> [_ w3314]
                  tunnel: w3307 -> [_ w3313]
                  tunnel: w3306 -> [_ w3312]
                  tunnel: w3305 -> [_ w3311]
                  frame False {
                  }
                  frame True {
                    n1769 = local read "DISP LAB05-2"() -> (w3310:T4)
                    n1770 = Unbundle(w3310) -> ("CYCLE"=w3318:dbl, "STATUS"=w3315:string)  [unwired: 1 out]
                    n1771 = global write "Global display 2.vi" "DISP LAB05-2"(w3310) -> ()
                    n1772 = Not Equal?(x=w3315, y="RUN") -> (x != y?=w3317:bool)
                    n1773 = local read "TDMS LAB05-2"() -> (w3321:refnum<k34>)
                    n1774 = Greater?(x=w3318, y=2.0) -> (0:w3319:bool)
                    n1775 = And(x=w3319, y=w3317) -> (x .and. y?=w3316:bool)
                    n1776 = case shown="True" w3316 {
                      tunnel: w3310 -> [_ w3329]
                      tunnel: w3321 -> [_ w3328]
                      tunnel: w3315 -> [_ w3327]
                      tunnel: w3314 -> [_ w3326]
                      tunnel: w3313 -> [_ w3325]
                      tunnel: w3312 -> [_ w3324]
                      tunnel: w3311 -> [_ w3323]
                      frame False {
                      }
                      frame True {
                        n1777 = stacked-sequence {
                          tunnel: w3329 -> [w3332 _ _]
                          tunnel: w3328 -> [_ w3334 _]
                          tunnel: w3327 -> [_ _ w3340]
                          tunnel: w3326 -> [_ _ w3339]
                          tunnel: w3325 -> [_ _ w3338]
                          tunnel: w3324 -> [_ _ w3337]
                          tunnel: w3323 -> [_ _ w3336]
                          frame #0 {
                            w3330 = FALSE
                            n1778 = local write "mail control"("END") -> ()
                            n1779 = Bundle(cluster=w3332) -> (w3333:T4)  [unwired: 3 in]
